vi "TEstConnect.vi"() -> ()   [LabVIEW 2019]
uses:
  D:/RLD_T14_2dScan/src/RF62X/RF62X-SDK/examples/LabVIEW/rf62Xsdk.dll
  rf62Xsdk.dll
panel:
  in  "file path":path
  out "XY Graph":cluster{sgl[], sgl[]}[](graph)
  out "Freq":dbl
  out "ProfPort":u16[](array[numeric])
  out "Disconnected":bool[](array[boolean])
  in  "stop":bool
  out "Npoints":i32
  out "Name":string[](array[string])
  out "Z":u32[](array[numeric])
  out "SdkInit":bool
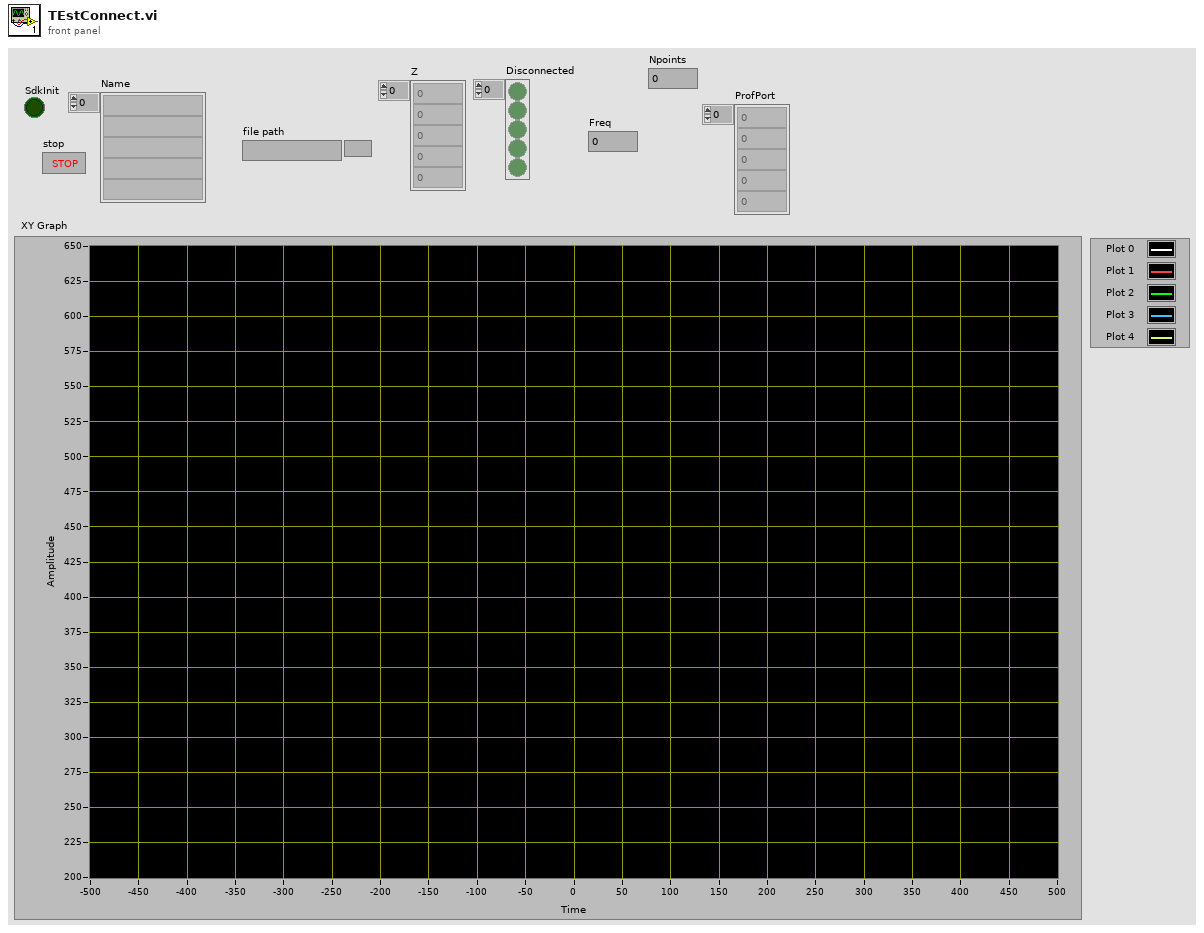
[diagram p1: front panel]
types:
  T1 = enum16{"open", "open or create", "create or replace", "create", "open (read-only)"}
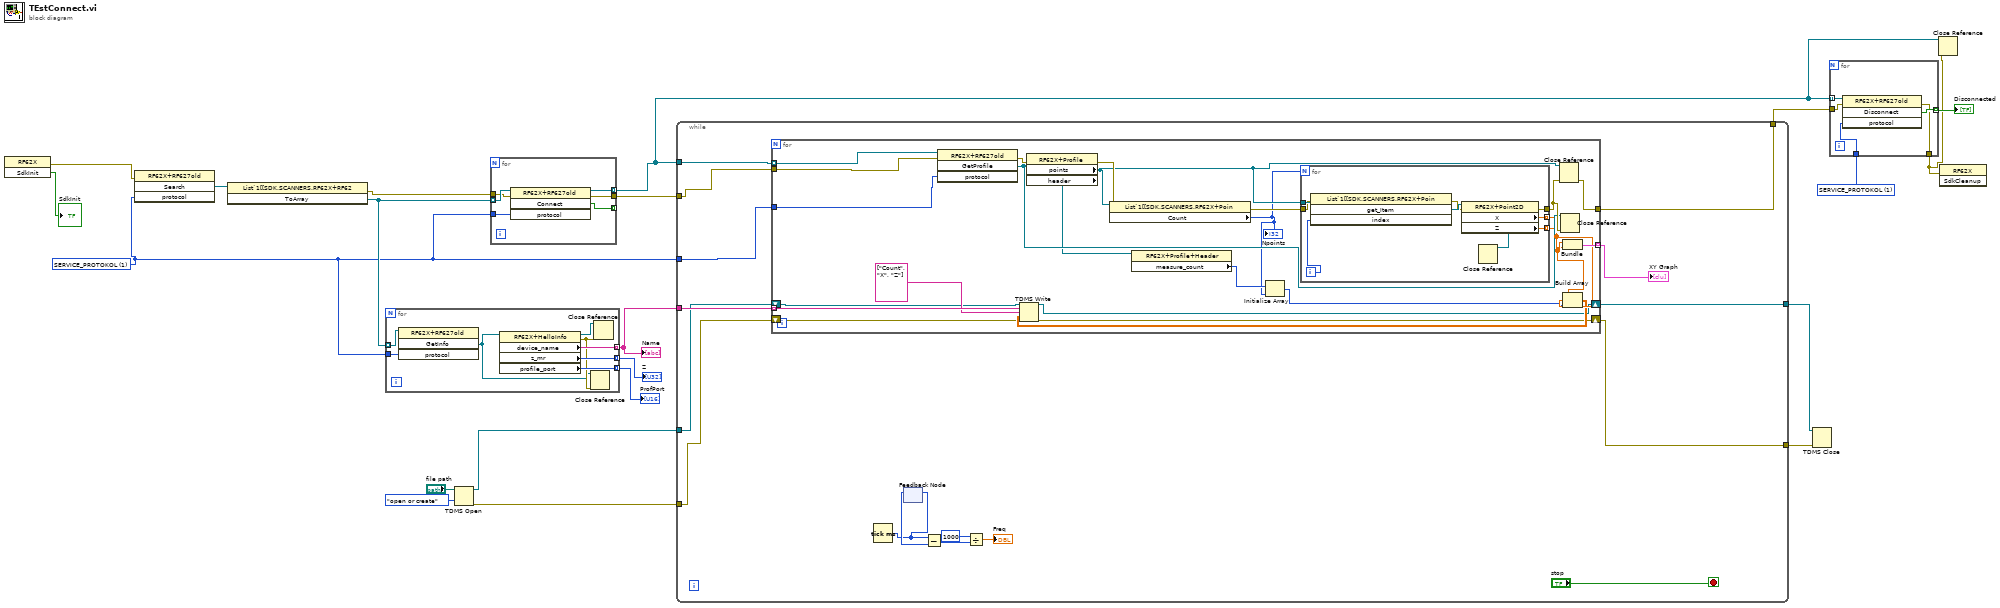
[diagram p0: block diagram]
diagram:
  w8 = 1 items=["SERVICE_PROTOKOL"=1, "ETHERNET_IP"=2, "MODBUS_TCP"=3] ("protocol")
  w9 = 1 items=["SERVICE_PROTOKOL"=1, "ETHERNET_IP"=2, "MODBUS_TCP"=3] ("protocol")
  n1 = invoke class="RF62X" method="SdkInit"() -> (error out=w19:errorcluster, "SdkInit"=→"SdkInit":bool)  [unwired: 3 in, 1 out]
  n2 = invoke class="RF62X+RF627old" method="Search"(error in=w19, "protocol"=w9) -> ("Search"=w20:refnum<k24>)  [unwired: 2 in, 3 out]
  n3 = invoke class="List`1[[SDK.SCANNERS.RF62X+RF62" method="ToArray"(reference=w20) -> (error out=w15:errorcluster, "ToArray"=w16:refnum<k24>[])  [unwired: 2 in, 1 out]
  n4 = for {
    tunnel: w16 -> [w25] mode=indexing
    tunnel: [w29] -> w3 mode=indexing
    tunnel: [w28] -> w18 mode=indexing
    tunnel: [w27] -> w17 mode=indexing
    tunnel: w9 -> [w26]
    n5 = invoke class="RF62X+RF627old" method="GetInfo"(reference=w25, "protocol"=w26) -> ("GetInfo"=w22:refnum<k24>)  [unwired: 2 in, 3 out]
    n6 = property class="RF62X+HelloInfo"(reference=w22) -> (reference out=w24:refnum<k24>, error out=w23:errorcluster, "device_name"=w29:string, "z_mr"=w28:u32, "profile_port"=w27:u16)  [unwired: 1 in]
    n7 = Close Reference(reference=w22, error in (no error)=w23) -> ()  [unwired: 1 out]
    n8 = Close Reference(reference=w24, error in (no error)=w23) -> ()  [unwired: 1 out]
  }
  "Z" <- w18
  "Name" <- w3
  "ProfPort" <- w17
  n9 = TDMS Open(10:T1."open or create" ("operation (0:open)"), 11:"file path") -> (0:w5:errorcluster, 3:w6:refnum<k34>)  [unwired: 5 in]
  n10 = for {
    tunnel: w16 -> [w35] mode=indexing
    tunnel: w15 -> [w34]
    tunnel: [w33] -> w13
    tunnel: [w32] -> w10 mode=indexing
    tunnel: [w31] -> _ mode=indexing
    tunnel: w9 -> [w30]
    n11 = invoke class="RF62X+RF627old" method="Connect"(reference=w35, error in=w34, "protocol"=w30) -> (reference out=w32:refnum<k24>, error out=w33:errorcluster, "Connect"=w31:bool)  [unwired: 1 in, 1 out]
  }
  n12 = while {
    tunnel: w9 -> [w51]
    tunnel: w13 -> [w44]
    tunnel: [w43] -> w12
    tunnel: w10 -> [w42]
    tunnel: w6 -> [w39]
    tunnel: w5 -> [w38]
    tunnel: w3 -> [w40]
    tunnel: [w37] -> w2
    tunnel: [w36] -> w1
    stop <- "stop" stop-if-true
    n13 = for {
      tunnel: w51 -> [w71]
      tunnel: w44 -> [w75]
      tunnel: [w65] -> w43
      tunnel: w42 -> [w72] mode=indexing
      tunnel: [w66] -> w41 mode=indexing
      tunnel: w40 -> [w58] mode=indexing
      shift-right: [w55] -> w36
      shift-left: w39 -> [w54]
      shift-right: [w53] -> w37
      shift-left: w38 -> [w52]
      n14 = invoke class="RF62X+RF627old" method="GetProfile"(reference=w72, error in=w75, "protocol"=w71) -> (error out=w74:errorcluster, "GetProfile"=w67:refnum<k24>)  [unwired: 1 in, 2 out]
      n15 = property class="RF62X+Profile"(reference=w67, error in=w74) -> (error out=w73:errorcluster, "points"=w69:refnum<k24>, "header"=w62:refnum<k24>)  [unwired: 1 out]
      n16 = property class="List`1[[SDK.SCANNERS.RF62X+Poin"(reference=w69, error in=w73) -> (error out=w70:errorcluster, "Count"=w60:i32)  [unwired: 1 out]
      "Npoints" <- w60
      n17 = property class="RF62X+Profile+Header"(reference=w62) -> ("measure_count"=w61:u32)  [unwired: 1 in, 2 out]
      n18 = Initialize Array(w61, w60) -> (w59:u32[])
      n19 = for {
        N: w60 -> [_]
        tunnel: w69 -> [w84]
        tunnel: [w81] -> w68
        tunnel: w70 -> [w80]
        tunnel: [w77] -> w64 mode=indexing
        tunnel: [w76] -> w63 mode=indexing
        i -> [w83]
        n20 = invoke class="List`1[[SDK.SCANNERS.RF62X+Poin" method="get_Item"(reference=w84, error in=w80, "index"=w83) -> (error out=w79:errorcluster, "get_Item"=w82:refnum<k24>)  [unwired: 1 in, 2 out]
        n21 = property class="RF62X+Point2D"(reference=w82, error in=w79) -> (reference out=w78:refnum<k24>, error out=w81:errorcluster, "X"=w77:sgl, "Z"=w76:sgl)
        n22 = Close Reference(reference=w78) -> ()  [unwired: 1 in, 1 out]
      }
      n23 = Close Reference(reference=w69, error in (no error)=w68) -> (error out=w65:errorcluster)
      n24 = Close Reference(reference=w67, error in (no error)=w68) -> ()  [unwired: 1 out]
      n25 = Bundle(w64, w63) -> (w66:cluster{sgl[], sgl[]})  [unwired: 1 in]
      n26 = Build Array(w64, w63, w59) -> (w56:sgl[][])
      n27 = TDMS Write(0:w54, 5:w58, 7:string[] ["Count", "X", "Z"] ("channel name(s) in (Untitled)"), 9:w56, 11:w52) -> (4:w55:refnum<k34>, 15:w53:errorcluster)  [unwired: 1 in, 2 out]
    }
    "XY Graph" <- w41
    n28 = Tick Count (ms)() -> (millisecond timer value=w46:u32)
    n29 = feedback-in #1(w46) -> ()
    n30 = feedback #1() -> (w50:u32)  [unwired: 1 in]
    n31 = Subtract(x=w46, y=w50) -> (x-y=w49:u32)
    n32 = Divide(x=u32 1000, y=w49) -> (x/y=→"Freq":dbl)
  }
  n33 = TDMS Close(8:w2, 11:w1) -> ()  [unwired: 2 out]
  n34 = for {
    tunnel: w10 -> [w89] mode=indexing
    tunnel: [w88] -> w14 mode=indexing
    tunnel: [w87] -> w11
    tunnel: w12 -> [w86]
    tunnel: w8 -> [w85]
    n35 = invoke class="RF62X+RF627old" method="Disconnect"(reference=w89, error in=w86, "protocol"=w85) -> (error out=w87:errorcluster, "Disconnect"=w88:bool)  [unwired: 1 in, 2 out]
  }
  "Disconnected" <- w14
  n36 = Close Reference(reference=w10, error in (no error)=w11) -> ()  [unwired: 1 out]
  n37 = invoke class="RF62X" method="SdkCleanup"(error in=w11) -> ()  [unwired: 2 in, 3 out]
